vi "Array(DBL)ToFile_v2_wrapper.vi"() -> ()   [LabVIEW 2014]
panel:
  out "data_string":string="25\r\n55\r\n73\r\n90\r\n25\r\n55\r\n73\r\n90\r\n25\r\n55\r\n73\r\n90\r\n25\r\n55\r\n73\r\n90\r\n25\r\n55\r\n73\r\n90\r\n25\r\n55\r\n73\r\n90\r\n25\r\n55\r\n73\r\n90\r\n25\r\n55\r\n73\r\n90\r\n25\r\n55\r\n73\r\n90\r\n25\r\n55\r\n73\r\n90\r\n25\r\n55\r\n73\r\n90\r\n25\r\n55\r\n73\r\n90\r\n25\r\n55\r\n73\r\n90\r\n25\r\n55\r\n73\r\n90\r\n25\r\n55\r\n73\r\n90\r\n25\r\n55\r\n73\r\n90\r\n25\r\n55\r\n73\r\n90\r\n25\r\n55\r\n73\r\n90\r\n25\r\n55\r\n73\r\n90\r\n25\r\n55\r\n73\r\n90\r\n25\r\n55\r\n73\r\n90\r\n25\r\n55\r\n73\r\n90\r\n25\r\n55\r\n73\r\n90\r\n25\r\n55\r\n73\r\n90\r\n25\r\n55\r\n73\r\n90\r\n25\r\n55\r\n73\r\n90\r\n25\r\n55\r\n73\r\n90\r\n25\r\n55\r\n73\r\n90\r\n25\r\n55\r\n73\r\n90\r\n25\r\n55\r\n73\r\n90\r\n25\r\n55\r\n73\r\n90\r\n25\r\n55\r\n73\r\n90\r\n25\r\n55\r\n73\r\n90\r\n25\r\n55\r\n73\r\n90\r\n25\r\n55\r\n73\r\n90\r\n25\r\n55\r\n73\r\n90\r\n25\r\n55\r\n73\r\n90\r\n25\r\n55\r\n..."
  out "Saved":bool=TRUE
  out "target_filepath":path=path "C:/misc/LabVIEW/FILES/SEQUENCES/OUT/seqOUT_trial01.psv"
  in  "Filename Collision Handling":T1(ring)
  in  "Parent Directory":path=path "C:/misc/LabVIEW/FILES"
  in  "data format (DBL)":string="%.8f"
  in  "delimiter (\"|\")":string="|"
  in  "Child Directory":path=path "SEQUENCES/OUT"
  in  "Array Type (2D)":enum16{"2D", "row", "column"}(ring)
  in  "2D-Array":dbl[][](array[numeric])=array100x100[10000 elements] format="%_8f"
  in  "1D-Array":dbl[](array[numeric])=[25.0, 55.0, 73.0, 90.0, 25.0, 55.0, 73.0, 90.0, 25.0, 55.0, 73.0, 90.0, 25.0, 55.0, 73.0, 90.0, 25.0, 55.0, 73.0, 90.0, 25.0, 55.0, 73.0, 90.0, 25.0, 55.0, 73.0, 90.0, 25.0, 55.0, 73.0, 90.0, 25.0, 55.0, 73.0, 90.0, 25.0, 55.0, 73.0, 90.0, 25.0, 55.0, 73.0, 90.0, 25.0, 55.0, 73.0, 90.0, 25.0, 55.0, 73.0, 90.0, 25.0, 55.0, 73.0, 90.0, 25.0, 55.0, 73.0, 90.0, 25.0, 55.0, 73.0, 90.0, 25.0, 55.0, 73.0, 90.0, 25.0, 55.0, 73.0, 90.0, 25.0, 55.0, 73.0, 90.0, 25.0, 55.0, 73.0, 90.0, 25.0, 55.0, 73.0, 90.0, 25.0, 55.0, 73.0, 90.0, 25.0, 55.0, 73.0, 90.0, 25.0, 55.0, 73.0, 90.0, 25.0, 55.0, 73.0, 90.0, 25.0, 55.0, 73.0, 90.0, 25.0, 55.0, 73.0, 90.0, 25.0, 55.0, 73.0, 90.0, 25.0, 55.0, 73.0, 90.0, 25.0, 55.0, 73.0, 90.0, 25.0, 55.0, 73.0, 90.0, 25.0, 55.0, 73.0, 90.0, 25.0, 55.0, 73.0, 90.0, 25.0, 55.0, 73.0, 90.0, 25.0, 55.0, 73.0, 90.0, 25.0, 55.0, 73.0, 90.0, 25.0, 55.0, 73.0, 90.0, 25.0, 55.0, 73.0, 90.0, 25.0, 55.0, 73.0, 90.0, 25.0, 55.0, 73.0, 90.0, 25.0, 55.0, 73.0, 90.0, 25.0, 55.0, 73.0, 90.0, 25.0, 55.0, 73.0, 90.0, 25.0, 55.0, 73.0, 90.0, 25.0, 55.0, 73.0, 90.0, 25.0, 55.0, 73.0, 90.0, 25.0, 55.0, 73.0, 90.0, 25.0, 55.0, 73.0, 90.0, 25.0, 55.0, 73.0, 90.0, 25.0, 55.0, 73.0, 90.0, 25.0, 55.0, 73.0, 90.0, 25.0, 55.0, 73.0, 90.0, 25.0, 55.0, 73.0, 90.0, 25.0, 55.0, 73.0, 90.0, 25.0, 55.0, 73.0, 90.0, 25.0, 55.0, 73.0, 90.0, 25.0, 55.0, 73.0, 90.0, 25.0, 55.0, 73.0, 90.0, 25.0, 55.0, 73.0, 90.0, 25.0, 55.0, 73.0, 90.0, 25.0, 55.0, 73.0, 90.0, 25.0, 55.0, 73.0, 90.0, 25.0, 55.0, 73.0, 90.0, 25.0, 55.0, 73.0, 90.0, 25.0, 55.0, 73.0, 90.0, 25.0, 55.0, 73.0, 90.0, 25.0, 55.0, 73.0, 90.0, 25.0, 55.0, 73.0, 90.0, 25.0, 55.0, 73.0, 90.0, 25.0, 55.0, 73.0, 90.0, 25.0, 55.0, 73.0, 90.0, 25.0, 55.0, 73.0, 90.0, 25.0, 55.0, 73.0, 90.0, 25.0, 55.0, 73.0, 90.0, 25.0, 55.0, 73.0, 90.0, 25.0, 55.0, 73.0, 90.0, 25.0, 55.0, 73.0, 90.0, 25.0, 55.0, 73.0, 90.0, 25.0, 55.0, 73.0, 90.0, 25.0, 55.0, 73.0, 90.0, 25.0, 55.0, 73.0, 90.0, 25.0, 55.0, 73.0, 90.0, 25.0, 55.0, 73.0, 90.0, 25.0, 55.0, 73.0, 90.0, 25.0, 55.0, 73.0, 90.0, 25.0, 55.0, 73.0, 90.0, 25.0, 55.0, 73.0, 90.0, 25.0, 55.0, 73.0, 90.0, 25.0, 55.0, 73.0, 90.0, 25.0, 55.0, 73.0, 90.0, 25.0, 55.0, 73.0, 90.0, 25.0, 55.0, 73.0, 90.0, 25.0, 55.0, 73.0, 90.0, 25.0, 55.0, 73.0, 90.0, 25.0, 55.0, 73.0, 90.0, 25.0, 55.0, 73.0, 90.0, 25.0, 55.0, 73.0, 90.0, 25.0, 55.0, 73.0, 90.0, 25.0, 55.0, 73.0, 90.0, 25.0, 55.0, 73.0, 90.0, 25.0, 55.0, 73.0, 90.0, 25.0, 55.0, 73.0, 90.0, 25.0, 55.0, 73.0, 90.0, 25.0, 55.0, 73.0, 90.0, 25.0, 55.0, 73.0, 90.0, 25.0, 55.0, 73.0, 90.0, 25.0, 55.0, 73.0, 90.0, 25.0, 55.0, 73.0, 90.0, 25.0, 55.0, 73.0, 90.0, 25.0, 55.0, 73.0, 90.0, 25.0, 55.0, 73.0, 90.0, 25.0, 55.0, 73.0, 90.0, 25.0, 55.0, 73.0, 90.0, 25.0, 55.0, 73.0, 90.0, 25.0, 55.0, 73.0, 90.0, 25.0, 55.0, 73.0, 90.0, 25.0, 55.0, 73.0, 90.0, 25.0, 55.0, 73.0, 90.0, 25.0, 55.0, 73.0, 90.0, 25.0, 55.0, 73.0, 90.0, 25.0, 55.0, 73.0, 90.0, 25.0, 55.0, 73.0, 90.0, 25.0, 55.0, 73.0, 90.0, 25.0, 55.0, 73.0, 90.0, 25.0, 55.0, 73.0, 90.0, 25.0, 55.0, 73.0, 90.0, 25.0, 55.0, 73.0, 90.0, 25.0, 55.0, 73.0, 90.0, 25.0, 55.0, 73.0, 90.0, 25.0, 55.0, 73.0, 90.0, 25.0, 55.0, 73.0, 90.0, 25.0, 55.0, 73.0, 90.0, 25.0, 55.0, 73.0, 90.0, 25.0, 55.0, 73.0, 90.0, 25.0, 55.0, 73.0, 90.0, 25.0, 55.0, 73.0, 90.0, 25.0, 55.0, 73.0, 90.0, 25.0, 55.0, 73.0, 90.0, 25.0, 55.0, 73.0, 90.0, 25.0, 55.0, 73.0, 90.0, 25.0, 55.0, 73.0, 90.0, 25.0, 55.0, 73.0, 90.0, 25.0, 55.0, 73.0, 90.0, 25.0, 55.0, 73.0, 90.0, 25.0, 55.0, 73.0, 90.0, 25.0, 55.0, 73.0, 90.0, 25.0, 55.0, 73.0, 90.0, 25.0, 55.0, 73.0, 90.0, 25.0, 55.0, 73.0, 90.0, 25.0, 55.0, 73.0, 90.0, 25.0, 55.0, 73.0, 90.0, 25.0, 55.0, 73.0, 90.0, 25.0, 55.0, 73.0, 90.0, 25.0, 55.0, 73.0, 90.0, 25.0, 55.0, 73.0, 90.0, 25.0, 55.0, 73.0, 90.0, 25.0, 55.0, 73.0, 90.0, 25.0, 55.0, 73.0, 90.0, 25.0, 55.0, 73.0, 90.0, 25.0, 55.0, 73.0, 90.0, 25.0, 55.0, 73.0, 90.0, 25.0, 55.0, 73.0, 90.0, 25.0, 55.0, 73.0, 90.0, 25.0, 55.0, 73.0, 90.0, 25.0, 55.0, 73.0, 90.0, 25.0, 55.0, 73.0, 90.0, 25.0, 55.0, 73.0, 90.0, 25.0, 55.0, 73.0, 90.0, 25.0, 55.0, 73.0, 90.0, 25.0, 55.0, 73.0, 90.0, 25.0, 55.0, 73.0, 90.0, 25.0, 55.0, 73.0, 90.0, 25.0, 55.0, 73.0, 90.0, 25.0, 55.0, 73.0, 90.0, 25.0, 55.0, 73.0, 90.0, 25.0, 55.0, 73.0, 90.0, 25.0, 55.0, 73.0, 90.0, 25.0, 55.0, 73.0, 90.0, 25.0, 55.0, 73.0, 90.0, 25.0, 55.0, 73.0, 90.0, 25.0, 55.0, 73.0, 90.0, 25.0, 55.0, 73.0, 90.0, 25.0, 55.0, 73.0, 90.0, 25.0, 55.0, 73.0, 90.0, 25.0, 55.0, 73.0, 90.0, 25.0, 55.0, 73.0, 90.0, 25.0, 55.0, 73.0, 90.0, 25.0, 55.0, 73.0, 90.0, 25.0, 55.0, 73.0, 90.0, 25.0, 55.0, 73.0, 90.0, 25.0, 55.0, 73.0, 90.0, 25.0, 55.0, 73.0, 90.0, 25.0, 55.0, 73.0, 90.0, 25.0, 55.0, 73.0, 90.0, 25.0, 55.0, 73.0, 90.0, 25.0, 55.0, 73.0, 90.0, 25.0, 55.0, 73.0, 90.0, 25.0, 55.0, 73.0, 90.0, 25.0, 55.0, 73.0, 90.0, 25.0, 55.0, 73.0, 90.0, 25.0, 55.0, 73.0, 90.0, 25.0, 55.0, 73.0, 90.0, 25.0, 55.0, 73.0, 90.0, 25.0, 55.0, 73.0, 90.0, 25.0, 55.0, 73.0, 90.0, 25.0, 55.0, 73.0, 90.0, 25.0, 55.0, 73.0, 90.0, 25.0, 55.0, 73.0, 90.0, 25.0, 55.0, 73.0, 90.0, 25.0, 55.0, 73.0, 90.0, 25.0, 55.0, 73.0, 90.0, 25.0, 55.0, 73.0, 90.0, 25.0, 55.0, 73.0, 90.0, 25.0, 55.0, 73.0, 90.0, 25.0, 55.0, 73.0, 90.0, 25.0, 55.0, 73.0, 90.0, 25.0, 55.0, 73.0, 90.0, 25.0, 55.0, 73.0, 90.0, 25.0, 55.0, 73.0, 90.0, 25.0, 55.0, 73.0, 90.0, 25.0, 55.0, 73.0, 90.0, 25.0, 55.0, 73.0, 90.0, 25.0, 55.0, 73.0, 90.0, 25.0, 55.0, 73.0, 90.0, 25.0, 55.0, 73.0, 90.0, 25.0, 55.0, 73.0, 90.0, 25.0, 55.0, 73.0, 90.0, 25.0, 55.0, 73.0, 90.0, 25.0, 55.0, 73.0, 90.0, 25.0, 55.0, 73.0, 90.0, 25.0, 55.0, 73.0, 90.0, 25.0, 55.0, 73.0, 90.0, 25.0, 55.0, 73.0, 90.0, 25.0, 55.0, 73.0, 90.0, 25.0, 55.0, 73.0, 90.0, 25.0, 55.0, 73.0, 90.0, 25.0, 55.0, 73.0, 90.0, 25.0, 55.0, 73.0, 90.0, 25.0, 55.0, 73.0, 90.0, 25.0, 55.0, 73.0, 90.0, 25.0, 55.0, 73.0, 90.0, 25.0, 55.0, 73.0, 90.0, 25.0, 55.0, 73.0, 90.0, 25.0, 55.0, 73.0, 90.0, 25.0, 55.0, 73.0, 90.0, 25.0, 55.0, 73.0, 90.0, 25.0, 55.0, 73.0, 90.0, 25.0, 55.0, 73.0, 90.0, 25.0, 55.0, 73.0, 90.0, 25.0, 55.0, 73.0, 90.0] format="%_8f"
  in  "extension (\".psv\")":string=".psv"
  in  "identifier(\"\")":string="trial01~000"
  in  "name_base":string="seqOUT"
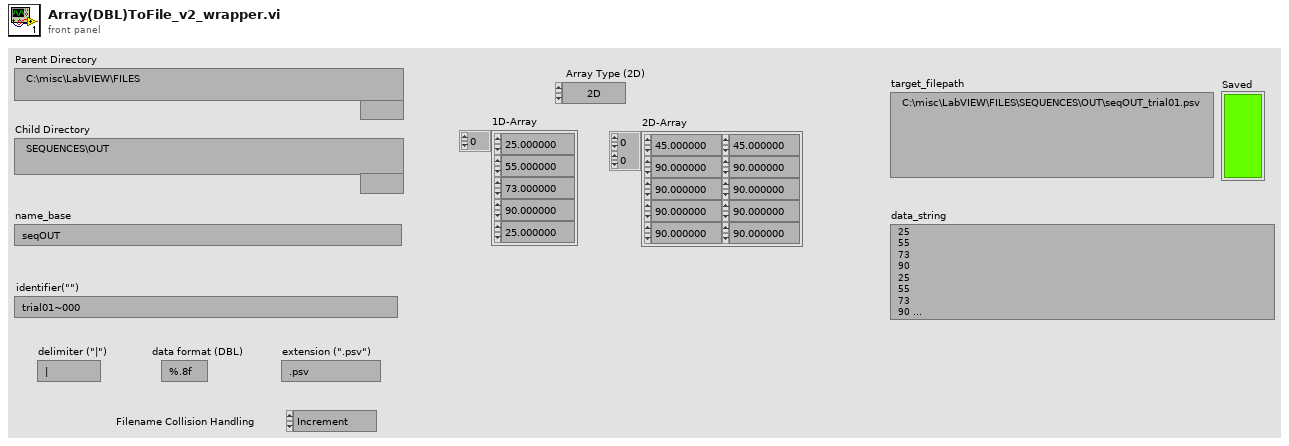
[diagram p1: front panel]
types:
  T1 = enum16{"Increment", "Overwrite", "Treat as Error"}
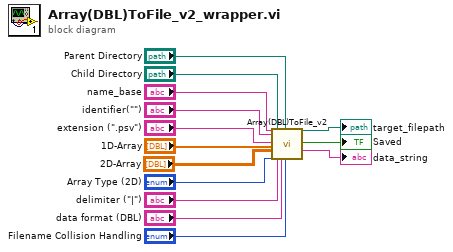
[diagram p0: block diagram]
diagram:
  n1 = call "Array(DBL)ToFile_v2.vi"("name_base"="name_base", "identifier(\"\")"="identifier(\"\")", "extension (\".psv\")"="extension (\".psv\")", "1D-Array"="1D-Array", "2D-Array"="2D-Array", "Array Type (2D)"="Array Type (2D)", "Child Directory"="Child Directory", "delimiter (\"|\")"="delimiter (\"|\")", "data format (DBL)"="data format (DBL)", "Parent Directory"="Parent Directory", "Filename Collision Handling"="Filename Collision Handling") -> ("target_filepath"=→"target_filepath":path, "Saved"=→"Saved":bool, "data_string"=→"data_string":string)  [unwired: 14 in]
